vi "ExecuteAux.vi"(7 "Intake Motor":T1={"DeviceStatus"={"status"=FALSE, "code"=0, "source"=""}, "Type"=enum."PWM", "PWM"={"PWM Channel"=enum."PWM 1", "DeadBand"={"Name"="", "maxPositivePwm"=0, "minPositivePwm"=0, "centerPwm"=0, "maxNegativePwm"=0, "minNegativePwm"=0, "angularRange"=0}}, "CAN"={"Device Number"=0, "SetOutput VI Ref"=variant(enum8{"Percent VBus", "Current", "Speed", "Position", "Voltage"} enum."Percent VBus"), "GetOutput VI Ref"=variant(refnum<k1> refnum), "Enable VI Ref"=variant(dbl 12.0), "Disable VI Ref"=variant(enum8{"Percent VBus", "Speed", "Position", "Slave", "Unchanged / Invalid", "Voltage Compensation", "Current", "Motion Profile"} enum."Percent VBus"), "Data"=variant}, "Invert"=FALSE, "DIO PWM"={"PWM \"Enable\" Channel"=enum."Invalid", "DIOChannel"=enum."Invalid", "PWM Rate"=0.0}}, 8 "error in":errorcluster, 9 "Belt Motor":T1={"DeviceStatus"={"status"=FALSE, "code"=0, "source"=""}, "Type"=enum."PWM", "PWM"={"PWM Channel"=enum."PWM 1", "DeadBand"={"Name"="", "maxPositivePwm"=0, "minPositivePwm"=0, "centerPwm"=0, "maxNegativePwm"=0, "minNegativePwm"=0, "angularRange"=0}}, "CAN"={"Device Number"=0, "SetOutput VI Ref"=variant(enum8{"Percent VBus", "Current", "Speed", "Position", "Voltage"} enum."Percent VBus"), "GetOutput VI Ref"=variant(refnum<k1> refnum), "Enable VI Ref"=variant(dbl 12.0), "Disable VI Ref"=variant(enum8{"Percent VBus", "Speed", "Position", "Slave", "Unchanged / Invalid", "Voltage Compensation", "Current", "Motion Profile"} enum."Percent VBus"), "Data"=variant}, "Invert"=FALSE, "DIO PWM"={"PWM \"Enable\" Channel"=enum."Invalid", "DIOChannel"=enum."Invalid", "PWM Rate"=0.0}}, 10 "Shooter Motor":T1={"DeviceStatus"={"status"=FALSE, "code"=0, "source"=""}, "Type"=enum."PWM", "PWM"={"PWM Channel"=enum."PWM 1", "DeadBand"={"Name"="", "maxPositivePwm"=0, "minPositivePwm"=0, "centerPwm"=0, "maxNegativePwm"=0, "minNegativePwm"=0, "angularRange"=0}}, "CAN"={"Device Number"=0, "SetOutput VI Ref"=variant(enum8{"Percent VBus", "Current", "Speed", "Position", "Voltage"} enum."Percent VBus"), "GetOutput VI Ref"=variant(refnum<k1> refnum), "Enable VI Ref"=variant(dbl 12.0), "Disable VI Ref"=variant(enum8{"Percent VBus", "Speed", "Position", "Slave", "Unchanged / Invalid", "Voltage Compensation", "Current", "Motion Profile"} enum."Percent VBus"), "Data"=variant}, "Invert"=FALSE, "DIO PWM"={"PWM \"Enable\" Channel"=enum."Invalid", "DIOChannel"=enum."Invalid", "PWM Rate"=0.0}}, 11 "Feeder Motor":T1={"DeviceStatus"={"status"=FALSE, "code"=0, "source"=""}, "Type"=enum."PWM", "PWM"={"PWM Channel"=enum."PWM 1", "DeadBand"={"Name"="", "maxPositivePwm"=0, "minPositivePwm"=0, "centerPwm"=0, "maxNegativePwm"=0, "minNegativePwm"=0, "angularRange"=0}}, "CAN"={"Device Number"=0, "SetOutput VI Ref"=variant(enum8{"Percent VBus", "Current", "Speed", "Position", "Voltage"} enum."Percent VBus"), "GetOutput VI Ref"=variant(refnum<k1> refnum), "Enable VI Ref"=variant(dbl 12.0), "Disable VI Ref"=variant(enum8{"Percent VBus", "Speed", "Position", "Slave", "Unchanged / Invalid", "Voltage Compensation", "Current", "Motion Profile"} enum."Percent VBus"), "Data"=variant}, "Invert"=FALSE, "DIO PWM"={"PWM \"Enable\" Channel"=enum."Invalid", "DIOChannel"=enum."Invalid", "PWM Rate"=0.0}}) -> (0 "error out":errorcluster)   [LabVIEW 2020]
uses:
  <vilib>/Rock Robotics/WPI/MotorControl/WPI_MotorControlDeviceRef.ctl
  <vilib>/Rock Robotics/WPI/MotorControl/WPI_MotorControlType.ctl
  <vilib>/Rock Robotics/SystemInterfaces/DIO/FPGA_DIOPWMChannel.ctl
  <vilib>/Rock Robotics/WPI/PWM/WPI_PWMDeadband.ctl
  <vilib>/Rock Robotics/SystemInterfaces/DIO/FPGA_DIOChannel.ctl
  <vilib>/Rock Robotics/WPI/ThirdParty/Phoenix-LabVIEW/Motor Controller/Controls/CTRE_Phoenix_MotorControl_ControlMode.ctl
  <vilib>/Rock Robotics/WPI/Solenoid/WPI_SolenoidValue.ctl
  <vilib>/Rock Robotics/WPI/ThirdParty/JAS_Junk/TrajLib/PIDController_AtSetpoint.vi
  <vilib>/Rock Robotics/WPI/ThirdParty/JAS_Junk/TrajLib/PIDController_SetPIDF.vi
  <vilib>/Rock Robotics/WPI/ThirdParty/JAS_Junk/TrajLib/PIDController_SetDerivativeFilter.vi
  <vilib>/Rock Robotics/WPI/ThirdParty/JAS_Junk/TrajLib/PIDController_SetIntegratorRange.vi
  <vilib>/Rock Robotics/WPI/ThirdParty/JAS_Junk/TrajLib/PIDController_SetTolerancePandV.vi
  <vilib>/Rock Robotics/WPI/ThirdParty/JAS_Junk/TrajLib/PIDController_DisableContinousInput.vi
  <vilib>/Rock Robotics/WPI/ThirdParty/JAS_Junk/TrajLib/PIDController_EnableContinousInput.vi
  <vilib>/Rock Robotics/WPI/ThirdParty/JAS_Junk/TrajLib/PIDController_Reset.vi
  <vilib>/Rock Robotics/WPI/ThirdParty/JAS_Junk/TrajLib/PIDController_New.vi
  <vilib>/Rock Robotics/WPI/ThirdParty/JAS_Junk/TrajLib/PIDController_SetOutputLimits.vi
  <vilib>/Rock Robotics/WPI/ThirdParty/JAS_Junk/TrajLib/SlewRateLimiter_New.vi
  <vilib>/Rock Robotics/WPI/ThirdParty/JAS_Junk/TrajLib/SlewRateLimiter_Reset.vi
  <vilib>/Rock Robotics/WPI/ThirdParty/JAS_Junk/TrajLib/SlewRateLimiter_Calculate.vi
  <vilib>/Rock Robotics/WPI/ThirdParty/JAS_Junk/TrajLib/SlewRateLimiter_SetRate.vi
  <vilib>/Rock Robotics/WPI/ThirdParty/JAS_Junk/TrajLib/ControllerUtil_GetModulusError.vi
  <vilib>/Rock Robotics/WPI/ThirdParty/JAS_Junk/TrajLib/PIDController_NewPeriod.vi
  <vilib>/Rock Robotics/SystemInterfaces/NetworkCommunication/NetComm_UsageReport_report.vi
  AuxGlobals.vi
  <vilib>/Rock Robotics/WPI/ThirdParty/JAS_Junk/TrajLib/Util_GetTime.vi
  <vilib>/Rock Robotics/WPI/ThirdParty/JAS_Junk/TrajLib/Util_LibraryGlobals.vi
  <vilib>/Rock Robotics/WPI/ThirdParty/JAS_Junk/TrajLib/PIDController_AdvCalculate_FF_Sp_Pv.vi
  <vilib>/Rock Robotics/WPI/Solenoid/WPI_SolenoidSetEnum.vi
  <vilib>/Rock Robotics/WPI/ThirdParty/JAS_Junk/TrajLib/Trajectory_Library.lvlib
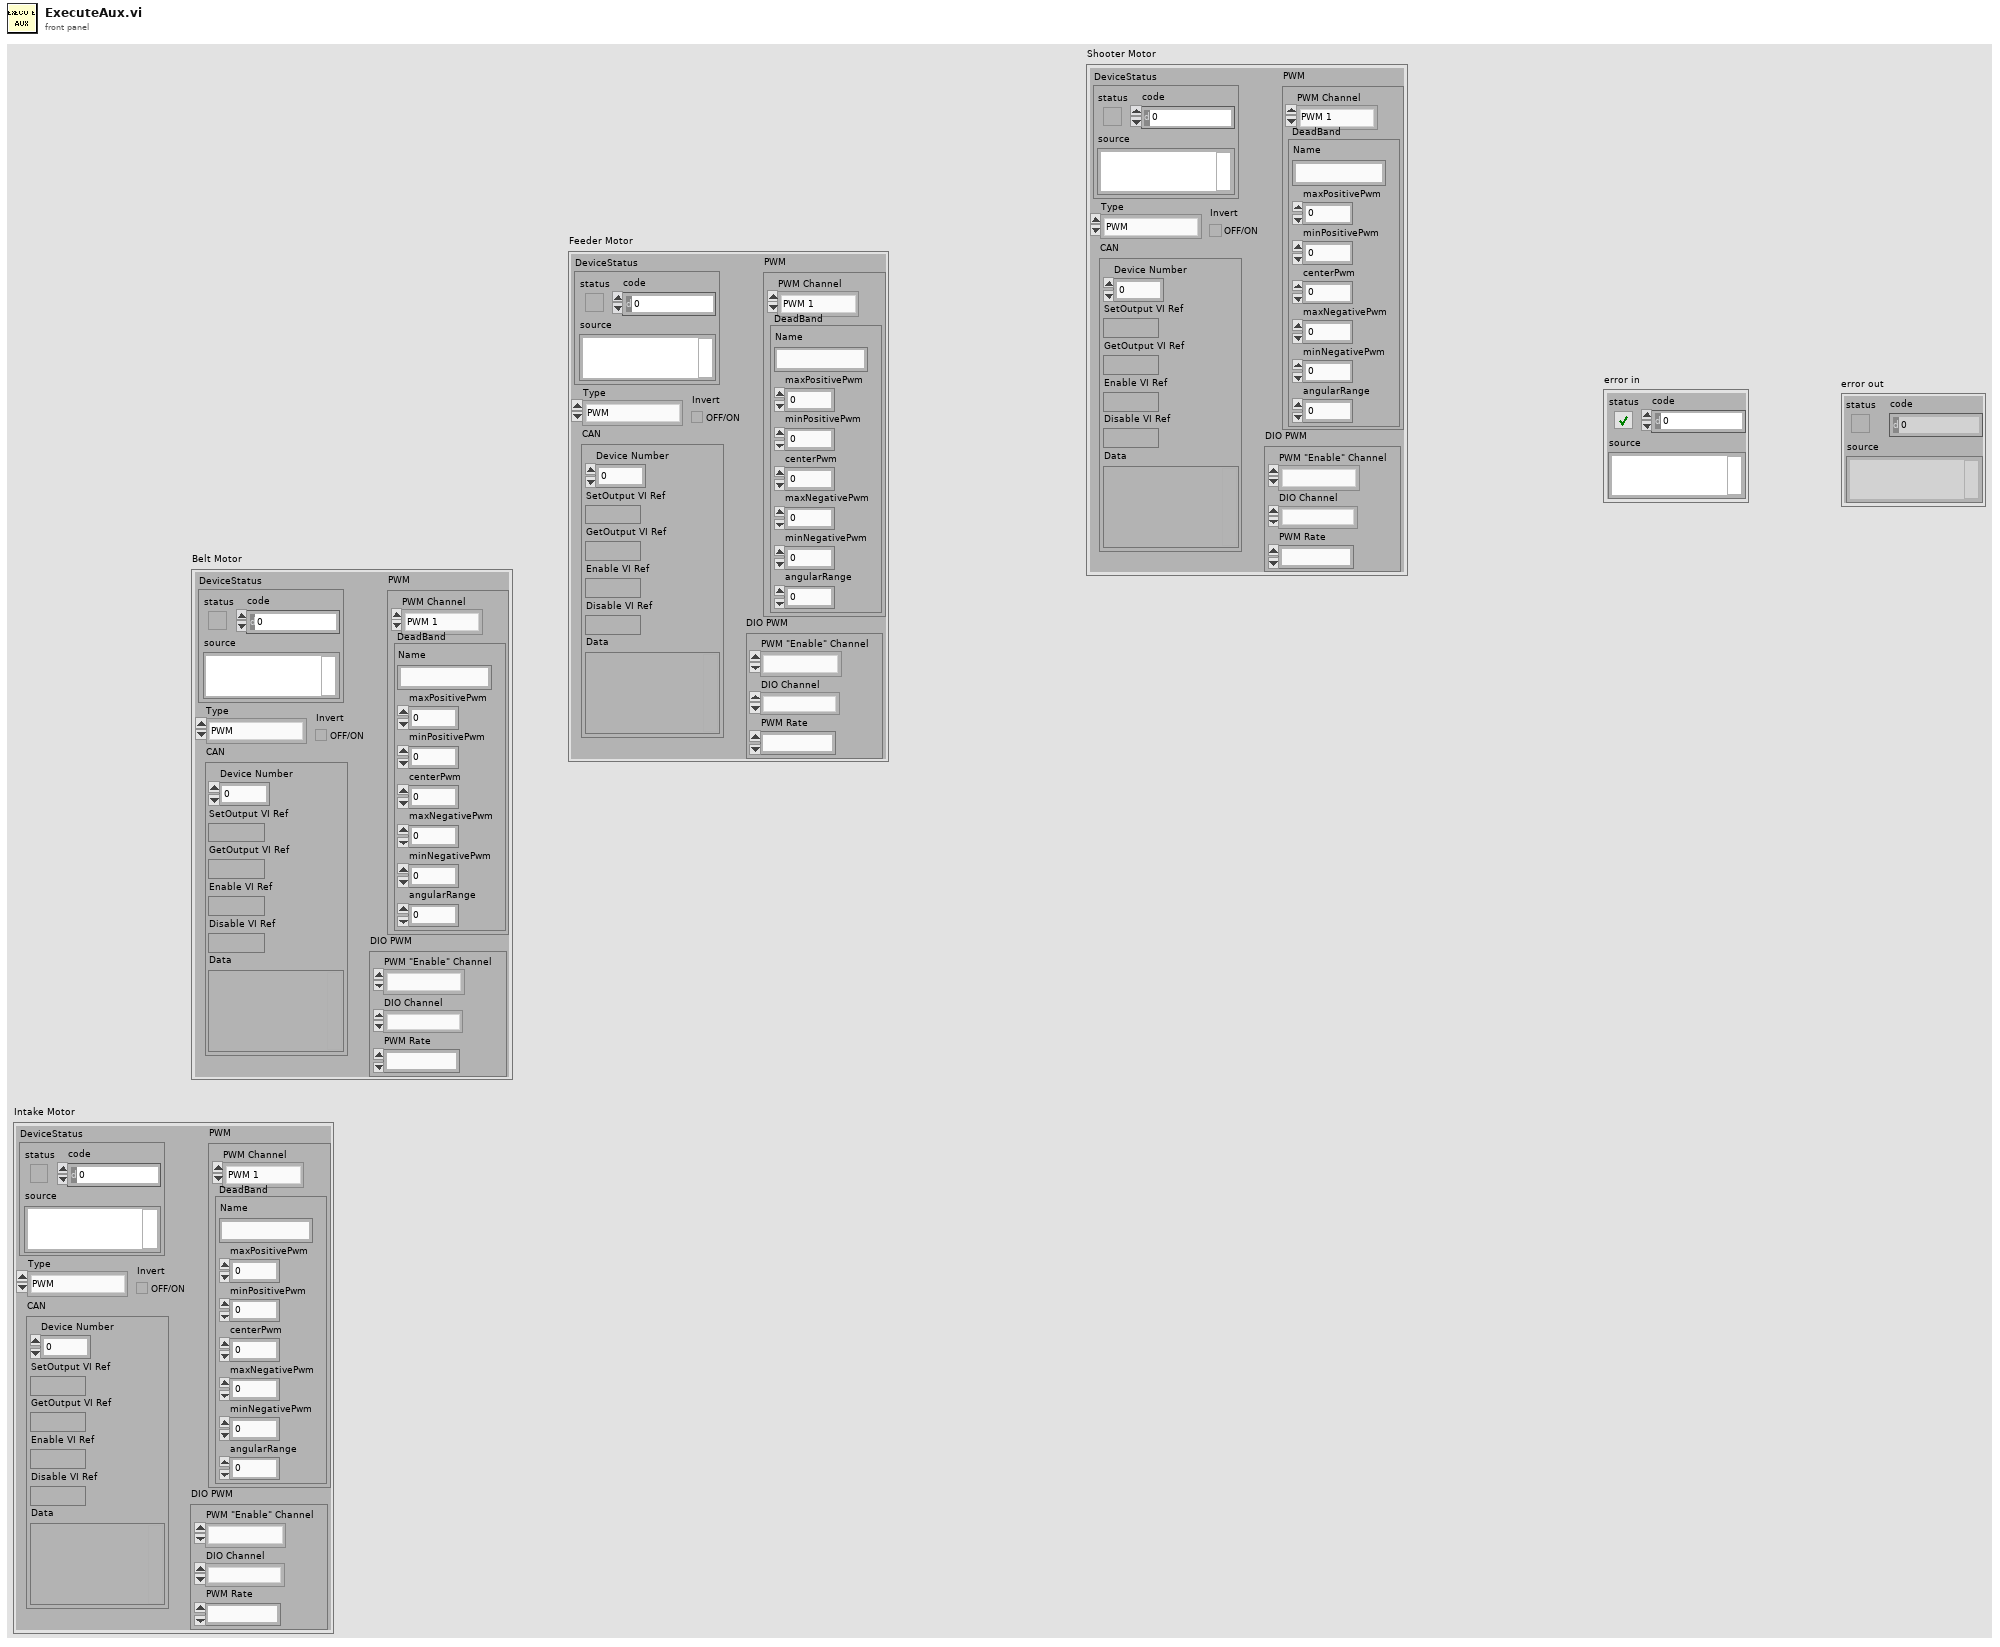
[diagram p1: front panel]
types:
  T1 = typedef "WPI_MotorControlDeviceRef.ctl" = cluster{"DeviceStatus":errorcluster, "Type":T2, "PWM":cluster{"PWM Channel":T3, "DeadBand":T4}, "CAN":cluster{"Device Number":u8, "SetOutput VI Ref":variant, "GetOutput VI Ref":variant, "Enable VI Ref":variant, "Disable VI Ref":variant, "Data":variant}, "Invert":bool, "DIO PWM":cluster{"PWM \"Enable\" Channel":T3, "DIOChannel":T5, "PWM Rate":dbl}}
  T2 = typedef "WPI_MotorControlType.ctl" = enum16{"PWM", "CAN", "DIO PWM"}
  T3 = typedef "FPGA_DIOPWMChannel.ctl" = enum8{"PWM 0", "PWM 1", "PWM 2", "PWM 3", "PWM 4", "PWM 5", "PWM 6", "PWM 7", "PWM 8", "PWM 9", "PWM MXP 0", "PWM MXP 1", "PWM MXP 2", "PWM MXP 3", "PWM MXP 4", "PWM MXP 5", "PWM MXP 6", "PWM MXP 7", "PWM MXP 8", "PWM MXP 9", "Invalid"}
  T4 = typedef "WPI_PWMDeadband.ctl" = cluster{"Name":string, "maxPositivePwm":i32, "minPositivePwm":i32, "centerPwm":i32, "maxNegativePwm":i32, "minNegativePwm":i32, "angularRange":u16}
  T5 = typedef "FPGA_DIOChannel.ctl" = enum8{"DIO 0", "DIO 1", "DIO 2", "DIO 3", "DIO 4", "DIO 5", "DIO 6", "DIO 7", "DIO 8", "DIO 9", "DIO MXP 0", "DIO MXP 1", "DIO MXP 2", "DIO MXP 3", "DIO MXP 4", "DIO MXP 5", "DIO MXP 6", "DIO MXP 7", "DIO MXP 8", "DIO MXP 9", "DIO MXP 10", "DIO MXP 11", "DIO MXP 12", "DIO MXP 13", "DIO MXP 14", "DIO MXP 15", "SPI Port CS1", "SPI Port CS2", "SPI Port CS3", "SPI Port MISO", "SPI Port MOSI", "Invalid"}
  T6 = typedef "CTRE_Phoenix_MotorControl_ControlMode.ctl" = u16
  T7 = typedef "WPI_SolenoidValue.ctl" = enum16{"Off", "On", "Forward", "Reverse"}
  T8 = typedef "WPI_SolenoidDevRef.ctl" = cluster{"DevStatus":errorcluster, "Pneumatics Control Module":u8, "Forward Solenoid Channel":T9, "Reverse Solenoid Channel":T9}
  T9 = typedef "WPI_SolenoidChannel.ctl" = enum8{"Solenoid 0", "Solenoid 1", "Solenoid 2", "Solenoid 3", "Solenoid 4", "Solenoid 5", "Solenoid 6", "Solenoid 7", "Solenoid 8", "Solenoid 9", "Solenoid 10", "Solenoid 11", "Solenoid 12", "Solenoid 13", "Solenoid 14", "Solenoid 15", "Invalid"}
  T10 = typedef "Trajectory_Library.lvlib/PID_ADV_LIMITS.ctl" = cluster{"MaxInput":dbl, "MinInput":dbl, "Continuous":bool, "MaxOutput":dbl, "MinOutput":dbl}
  T11 = typedef "Trajectory_Library.lvlib/PID_ADV_TUNING.ctl" = cluster{"Kf":dbl, "Kp":dbl, "Ki":dbl, "Kd":dbl, "MaximumIntegral":dbl, "MinimumIntegral":dbl, "Filter Derivative":bool}
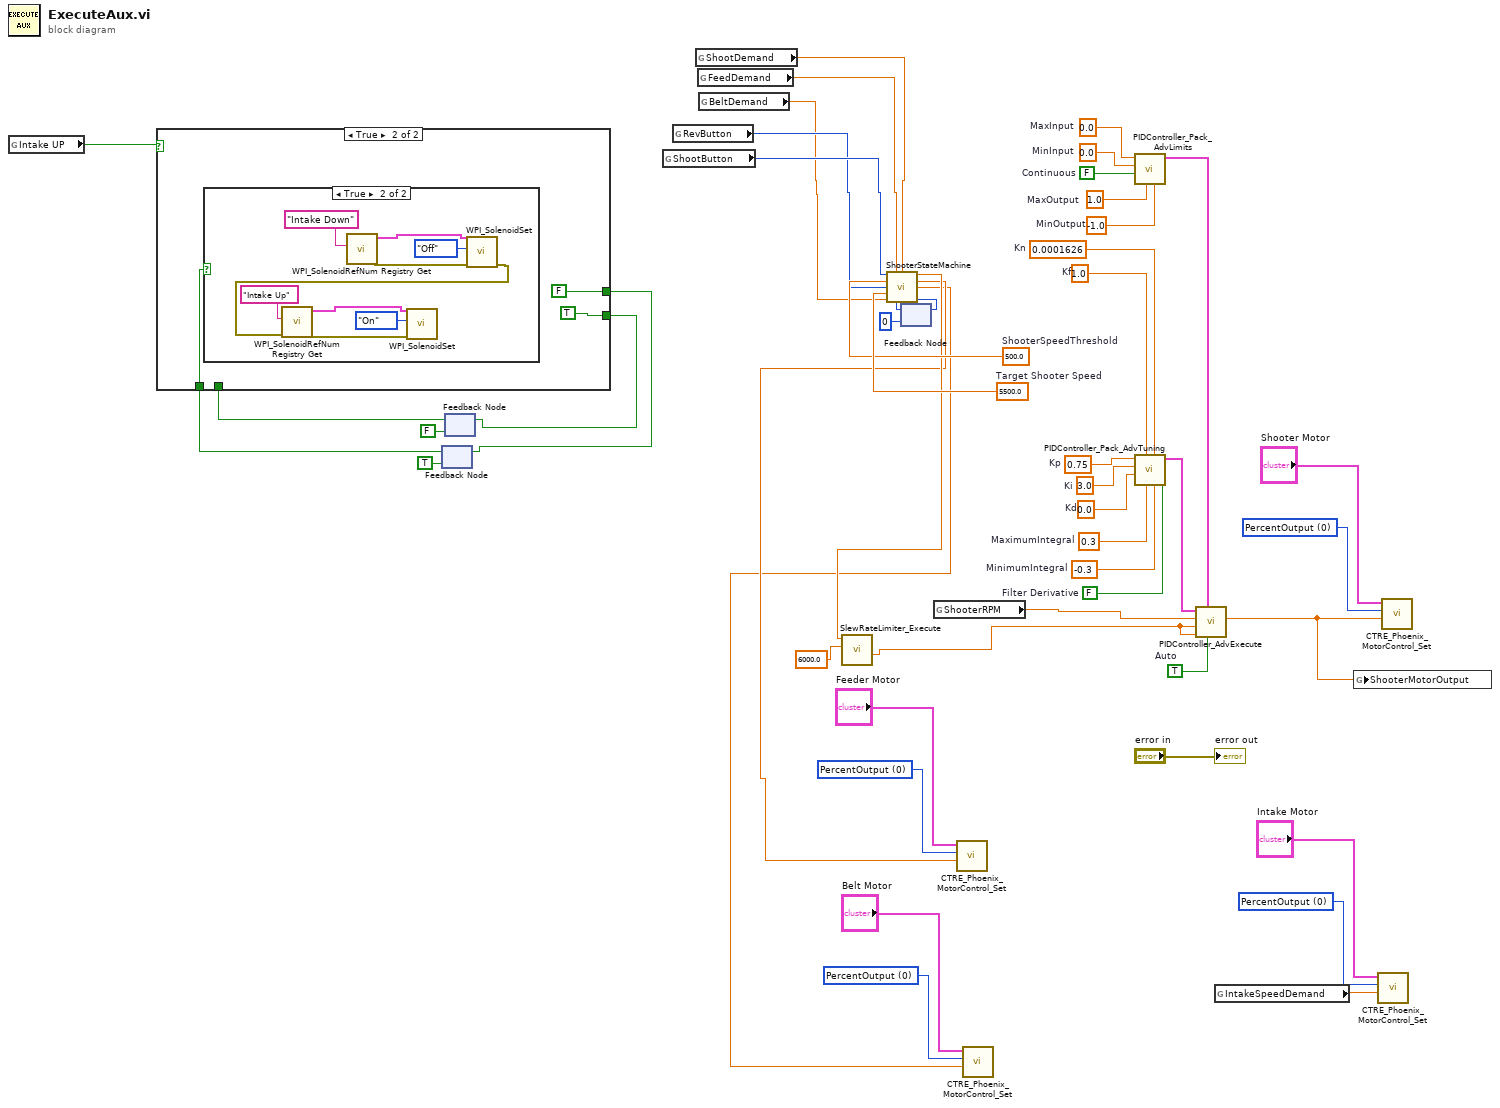
[diagram p0: block diagram]
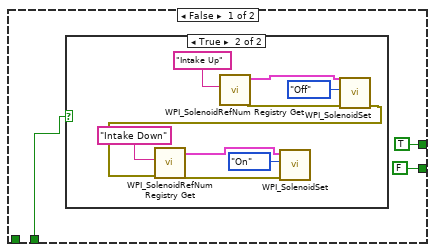
[diagram p2: hidden frame]
diagram:
  w9 = 500.0  # ShooterSpeedThreshold
  w10 = 5500.0  # Target Shooter Speed
  w22 = T6 0 items=["PercentOutput"=0, "Position"=1, "Velocity"=2, "Current"=3, "Follower"=5, "MotionProfile"=6, "MotionMagic"=7, "MotionProfileArc"=10, "Disabled"=15] ("Control Mode")
  w24 = T6 0 items=["PercentOutput"=0, "Position"=1, "Velocity"=2, "Current"=3, "Follower"=5, "MotionProfile"=6, "MotionMagic"=7, "MotionProfileArc"=10, "Disabled"=15] ("Control Mode")
  w26 = T6 0 items=["PercentOutput"=0, "Position"=1, "Velocity"=2, "Current"=3, "Follower"=5, "MotionProfile"=6, "MotionMagic"=7, "MotionProfileArc"=10, "Disabled"=15] ("Control Mode")
  w31 = T6 0 items=["PercentOutput"=0, "Position"=1, "Velocity"=2, "Current"=3, "Follower"=5, "MotionProfile"=6, "MotionMagic"=7, "MotionProfileArc"=10, "Disabled"=15] ("Control Mode")
  w34 = TRUE  # Auto
  w49 = 0.0001626  # Kn
  w48 = 0.75  # Kp
  w47 = 3.0  # Ki
  w46 = 0.0  # Kd
  w45 = 1.0  # Kf
  w44 = 0.3  # MaximumIntegral
  w43 = -0.3  # MinimumIntegral
  w42 = FALSE  # Filter Derivative
  w40 = 0.0  # MinInput
  w39 = FALSE  # Continuous
  w38 = 1.0  # MaxOutput
  w41 = -1.0  # MinOutput
  w37 = 0.0  # MaxInput
  n1 = global read "AuxGlobals.vi" "Intake UP"() -> (w20:bool)
  n2 = feedback #1(TRUE) -> (w19:bool)
  n3 = feedback #2(FALSE) -> (w14:bool)
  n4 = case shown="True" w20 {
    tunnel: w19 -> [_ w64]
    tunnel: [TRUE FALSE] -> w18
    tunnel: [FALSE TRUE] -> w15
    tunnel: w14 -> [w51 _]
    frame False {
      n5 = case shown="True" w51 {
        frame False {
        }
        frame True {
          n6 = call <vilib>:"WPI_SolenoidRefNum Registry Get.vi"("refnum name"="Intake Up") -> ("error out"=w62:errorcluster, "SolenoidDevRef"=w54:T8)  [unwired: 9 in]
          n7 = call-poly <vilib>:"WPI_SolenoidSet.vi"("error in (no error)"=w62, "Value"=WPI_SolenoidValue."Off", "SolenoidDevRef"=w54) -> ("error out"=w61:errorcluster)  [unwired: 7 in, 1 out]
          n8 = call <vilib>:"WPI_SolenoidRefNum Registry Get.vi"("error in (no error)"=w61, "refnum name"="Intake Down") -> ("error out"=w60:errorcluster, "SolenoidDevRef"=w55:T8)  [unwired: 8 in]
          n9 = call-poly <vilib>:"WPI_SolenoidSet.vi"("error in (no error)"=w60, "Value"=WPI_SolenoidValue."On", "SolenoidDevRef"=w55) -> ()  [unwired: 7 in, 2 out]
        }
      }
    }
    frame True {
      n10 = case shown="True" w64 {
        frame False {
        }
        frame True {
          n11 = call <vilib>:"WPI_SolenoidRefNum Registry Get.vi"("refnum name"="Intake Down") -> ("error out"=w68:errorcluster, "SolenoidDevRef"=w67:T8)  [unwired: 9 in]
          n12 = call-poly <vilib>:"WPI_SolenoidSet.vi"("error in (no error)"=w68, "Value"=WPI_SolenoidValue."Off", "SolenoidDevRef"=w67) -> ("error out"=w69:errorcluster)  [unwired: 7 in, 1 out]
          n13 = call <vilib>:"WPI_SolenoidRefNum Registry Get.vi"("error in (no error)"=w69, "refnum name"="Intake Up") -> ("error out"=w70:errorcluster, "SolenoidDevRef"=w66:T8)  [unwired: 8 in]
          n14 = call-poly <vilib>:"WPI_SolenoidSet.vi"("error in (no error)"=w70, "Value"=WPI_SolenoidValue."On", "SolenoidDevRef"=w66) -> ()  [unwired: 7 in, 2 out]
        }
      }
    }
  }
  n15 = feedback-in #1(w18) -> ()
  n16 = feedback-in #2(w15) -> ()
  n17 = global read "AuxGlobals.vi" "ShootButton"() -> (w6:i64)
  n18 = global read "AuxGlobals.vi" "RevButton"() -> (w5:i64)
  n19 = global read "AuxGlobals.vi" "ShootDemand"() -> (w8:dbl)
  n20 = global read "AuxGlobals.vi" "FeedDemand"() -> (w7:dbl)
  n21 = global read "AuxGlobals.vi" "BeltDemand"() -> (w4:dbl)
  n22 = feedback #3(0 ("NextState")) -> (w12:i32)
  n23 = call "ShooterStateMachine.vi"("Shoot Button"=w6, "FeederSpeedDemand"=w7, "ShooterSpeedDemand"=w8, "ShooterSpeedThreshold"=w9, "Rev Button"=w5, "Target Shooter Speed"=w10, "BeltSpeedDemand"=w4, "State"=w12) -> ("ShooterSpeed"=w3:dbl, "FeederSpeed"=w2:dbl, "BeltSpeed"=w1:dbl, "NextState"=w13:i32)  [unwired: 4 in]
  n24 = call <vilib>:"SlewRateLimiter_Execute.vi"("Rate"=6000.0, "Input"=w3) -> ("Output"=w30:dbl)  [unwired: 8 in, 1 out]
  n25 = feedback-in #3(w13) -> ()
  n26 = global read "AuxGlobals.vi" "ShooterRPM"() -> (w33:dbl)
  n27 = call <vilib>:"CTRE_Phoenix_MotorControl_Set.vi"("Output"=w2, "Control Mode"=w26, "PhoenixMotorControlDevRef"="Feeder Motor") -> ()  [unwired: 7 in, 2 out]
  n28 = call <vilib>:"CTRE_Phoenix_MotorControl_Set.vi"("Output"=w1, "Control Mode"=w24, "PhoenixMotorControlDevRef"="Belt Motor") -> ()  [unwired: 7 in, 2 out]
  n29 = call <vilib>:"PIDController_Pack_AdvLimits.vi"("MinOutput"=w41, "MaxOutput"=w38, "Continuous"=w39, "MinInput"=w40, "MaxInput"=w37) -> ("Adv PID Limits"=w35:T10)  [unwired: 6 in]
  n30 = call <vilib>:"PIDController_Pack_AdvTuning.vi"("Filter Derivative"=w42, "MinimumIntegral"=w43, "Kn"=w49, "MaximumIntegral"=w44, "Kf"=w45, "Kd"=w46, "Ki"=w47, "Kp"=w48) -> ("Adv PID Tuning"=w36:T11)  [unwired: 3 in]
  n31 = call <vilib>:"PIDController_AdvExecute.vi"("Auto"=w34, "Adv PID Limits"=w35, "FF-FeedForward"=w30, "SP-SetPoint"=w30, "PV-Measurement"=w33, "Adv PID Tuning"=w36) -> ("CO-ControlOutput"=w29:dbl)  [unwired: 3 in, 2 out]
  n32 = global read "AuxGlobals.vi" "IntakeSpeedDemand"() -> (w21:dbl)
  n33 = global write "AuxGlobals.vi" "ShooterMotorOutput"(w29) -> ()
  n34 = call <vilib>:"CTRE_Phoenix_MotorControl_Set.vi"("Output"=w21, "Control Mode"=w22, "PhoenixMotorControlDevRef"="Intake Motor") -> ()  [unwired: 7 in, 2 out]
  n35 = call <vilib>:"CTRE_Phoenix_MotorControl_Set.vi"("Output"=w29, "Control Mode"=w31, "PhoenixMotorControlDevRef"="Shooter Motor") -> ()  [unwired: 7 in, 2 out]
  "error out" <- "error in"
